vi "CS++CoreGUIContent.vi"() -> (0 "CS++Classes & Messages":T1(array[cluster]))   [LabVIEW 2015]
doc: "Place actor and class constants that should be included included in an application on the blockdiagramm."
uses:
  <vilib>/ActorFramework/Message/Message.lvclass
  Actors/CS++GUIActor/CS++GUIActor.lvclass
  Actors/CS++DeviceGUIActor/CS++DeviceGUIActor.lvclass
  Actors/CS++BaseActor/CS++BaseActor.lvclass
panel:
  # "Place actor and class constants on the blockdiagramm."
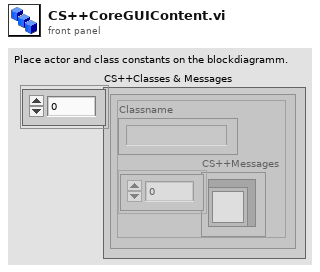
[diagram p1: front panel]
types:
  T1 = cluster{"Classname":string, "CS++Messages":refnum<class "Message.lvclass">[]}[]
  T2 = cluster{"class name":string, "CS++Messages":refnum<class "Message.lvclass">[]}
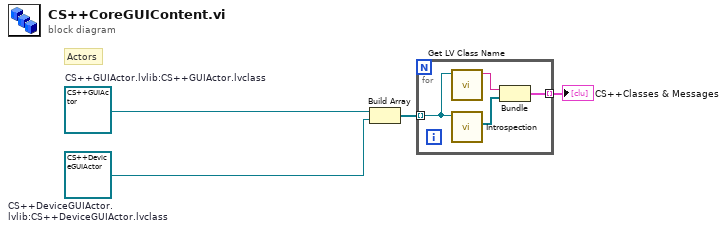
[diagram p0: block diagram]
diagram:
  w2 = refnum<class "CS++DeviceGUIActor.lvclass"> refnum  # CS++DeviceGUIActor.lvlib:CS++DeviceGUIActor.lvclass
  w3 = refnum<class "CS++GUIActor.lvclass"> refnum  # CS++GUIActor.lvlib:CS++GUIActor.lvclass
  # "Actors"
  n1 = Build Array(w3, w2) -> (w1:refnum<class "CS++GUIActor.lvclass">[])
  n2 = for {
    tunnel: w1 -> [w8] mode=indexing
    tunnel: [w5] -> w4 mode=indexing
    n3 = call <vilib>:"Get LV Class Name.vi"("object"=w8) -> ("class name"=w7:string)  [unwired: 9 in, 1 out]
    n4 = call "Introspection.vi"("CS++BaseActor in"=w8) -> ("CS++Messages"=w6:refnum<class "Message.lvclass">[])  [unwired: 8 in, 2 out]
    n5 = Bundle("class name"=w7, "CS++Messages"=w6) -> (w5:T2)  [unwired: 1 in]
  }
  "CS++Classes & Messages" <- w4
